vi "last data.vi"(8 "data interval":sgl format="%.2f", 11 "calibrated data":sgl[][](array[numeric]) format="%.5f") -> (0 "last reading":sgl[](array[numeric]) format="%.2f", 1 "first derivative":sgl[](array[numeric]) format="%.2f")   [LabVIEW 2012]
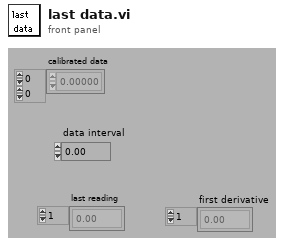
[diagram p1: front panel]
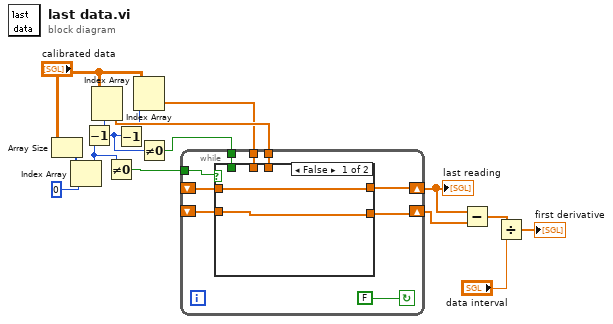
[diagram p0: block diagram]
diagram:
  n1 = Array Size(array="calibrated data") -> (size(s)=w14:i32[])
  n2 = Index Array(array=w14, index=0) -> (element=w13:i32)
  n3 = Decrement(x=w13) -> (x-1=w8:i32)
  n4 = Index Array(array="calibrated data", index (row)=w8) -> (element=w11:sgl[])  [unwired: 1 in]
  n5 = Not Equal To 0?(x=w13) -> (x != 0?=w12:bool)
  n6 = Decrement(x=w8) -> (x-1=w9:i32)
  n7 = Index Array(array="calibrated data", index (row)=w9) -> (element=w6:sgl[])  [unwired: 1 in]
  n8 = Not Equal To 0?(x=w8) -> (x != 0?=w7:bool)
  n9 = while {
    tunnel: w6 -> [w18]
    tunnel: w7 -> [w20]
    shift-left: _ -> [w17]
    shift-right: [w19] -> w4
    tunnel: w11 -> [w22]
    tunnel: w12 -> [w24]
    shift-left: _ -> [w21]
    shift-right: [w23] -> w5
    stop <- FALSE continue-if-true
    n10 = case shown="False" w24 {
      tunnel: [w26 w31] -> w23
      tunnel: w22 -> [_ w31]
      tunnel: w21 -> [w26 w27]
      tunnel: w20 -> [_ w30]
      tunnel: [w25 w29] -> w19
      tunnel: w18 -> [_ w28]
      tunnel: w17 -> [w25 _]
      frame False {
      }
      frame True {
        n11 = case shown="False" w30 {
          tunnel: [w32 w33] -> w29
          tunnel: w28 -> [_ w33]
          tunnel: w27 -> [w32 _]
          frame False {
          }
          frame True {
          }
        }
      }
    }
  }
  "last reading" <- w5
  n12 = Subtract(x=w5, y=w4) -> (x-y=w3:sgl[])
  n13 = Divide(x=w3, y="data interval") -> (x/y=→"first derivative":sgl[])
